vi "Spline_getPoint.vi"(8 "inputSPLINE":T1, 11 "Time":dbl) -> (3 "POSEwCURVATURE":T3={"CURVATURE"=0.0, "POSE"={"TRANSLATION"={"X"=0.0, "Y"=0.0}, "ROTATION"={"VALUE"=0.0, "COS"=1.0, "SIN"=0.0}}} {"POSE"."ROTATION"."SIN" format="%13.4f"; "POSE"."ROTATION"."COS" format="%13.4f"; "POSE"."ROTATION"."VALUE" format="%13.4f"; "POSE"."TRANSLATION"."Y" format="%14.3f"; "POSE"."TRANSLATION"."X" format="%14.3f"})   [LabVIEW 2019, in "Trajectory_Library.lvlib"]
doc: "Gets the pose and curvature at some point t on the spline.\n\nParameters:\n - Input Spline - Spline data structure\n - Time - The point in time to evaluate. (between 0 and 1)\n\nReturns:\n - PoseWCurve - The pose and curvature at that point."
uses:
  Trajectory_Library.lvlib
  TypeDef/POSEwCURVATURE.ctl
  TypeDef/POSE2D.ctl
  TypeDef/TRANSLATION2D.ctl
  TypeDef/ROTATION2D.ctl
  TypeDef/SPLINE.ctl
  <vilib>/Analysis/Matrix/Datatypes/RealMatrix.ctl
  <vilib>/Analysis/Matrix/Numeric/Multiply/Multiply - RM,RM.vi
  <vilib>/Analysis/Matrix/NI_Matrix.lvlib
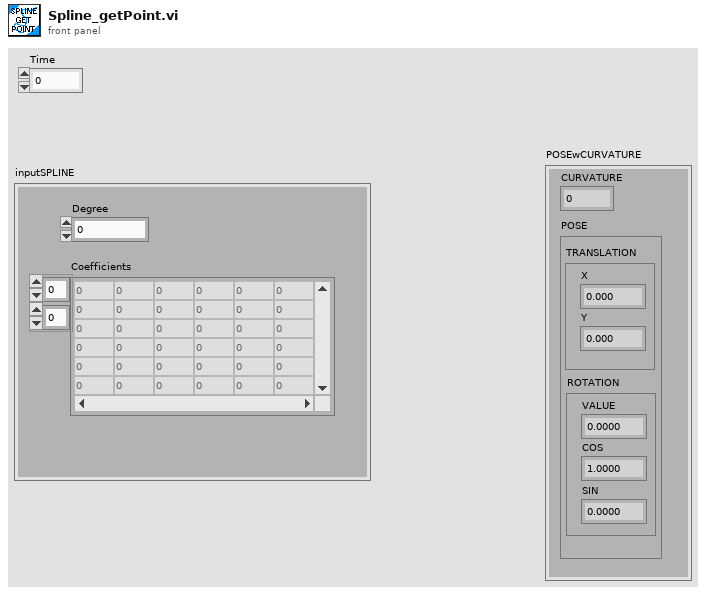
[diagram p1: front panel]
types:
  T1 = typedef "Trajectory_Library.lvlib/SPLINE.ctl" = cluster{"Degree":i32, "Coefficients":T2}
  T2 = typedef "NI_Matrix.lvlib/RealMatrix.ctl" = dbl[][]
  T3 = typedef "Trajectory_Library.lvlib/POSEwCURVATURE.ctl" = cluster{"CURVATURE":dbl, "POSE":T4}
  T4 = typedef "Trajectory_Library.lvlib/POSE2D.ctl" = cluster{"TRANSLATION":T5, "ROTATION":T6}
  T5 = typedef "Trajectory_Library.lvlib/TRANSLATION2D.ctl" = cluster{"X":dbl, "Y":dbl}
  T6 = typedef "Trajectory_Library.lvlib/ROTATION2D.ctl" = cluster{"VALUE":dbl, "COS":dbl, "SIN":dbl}
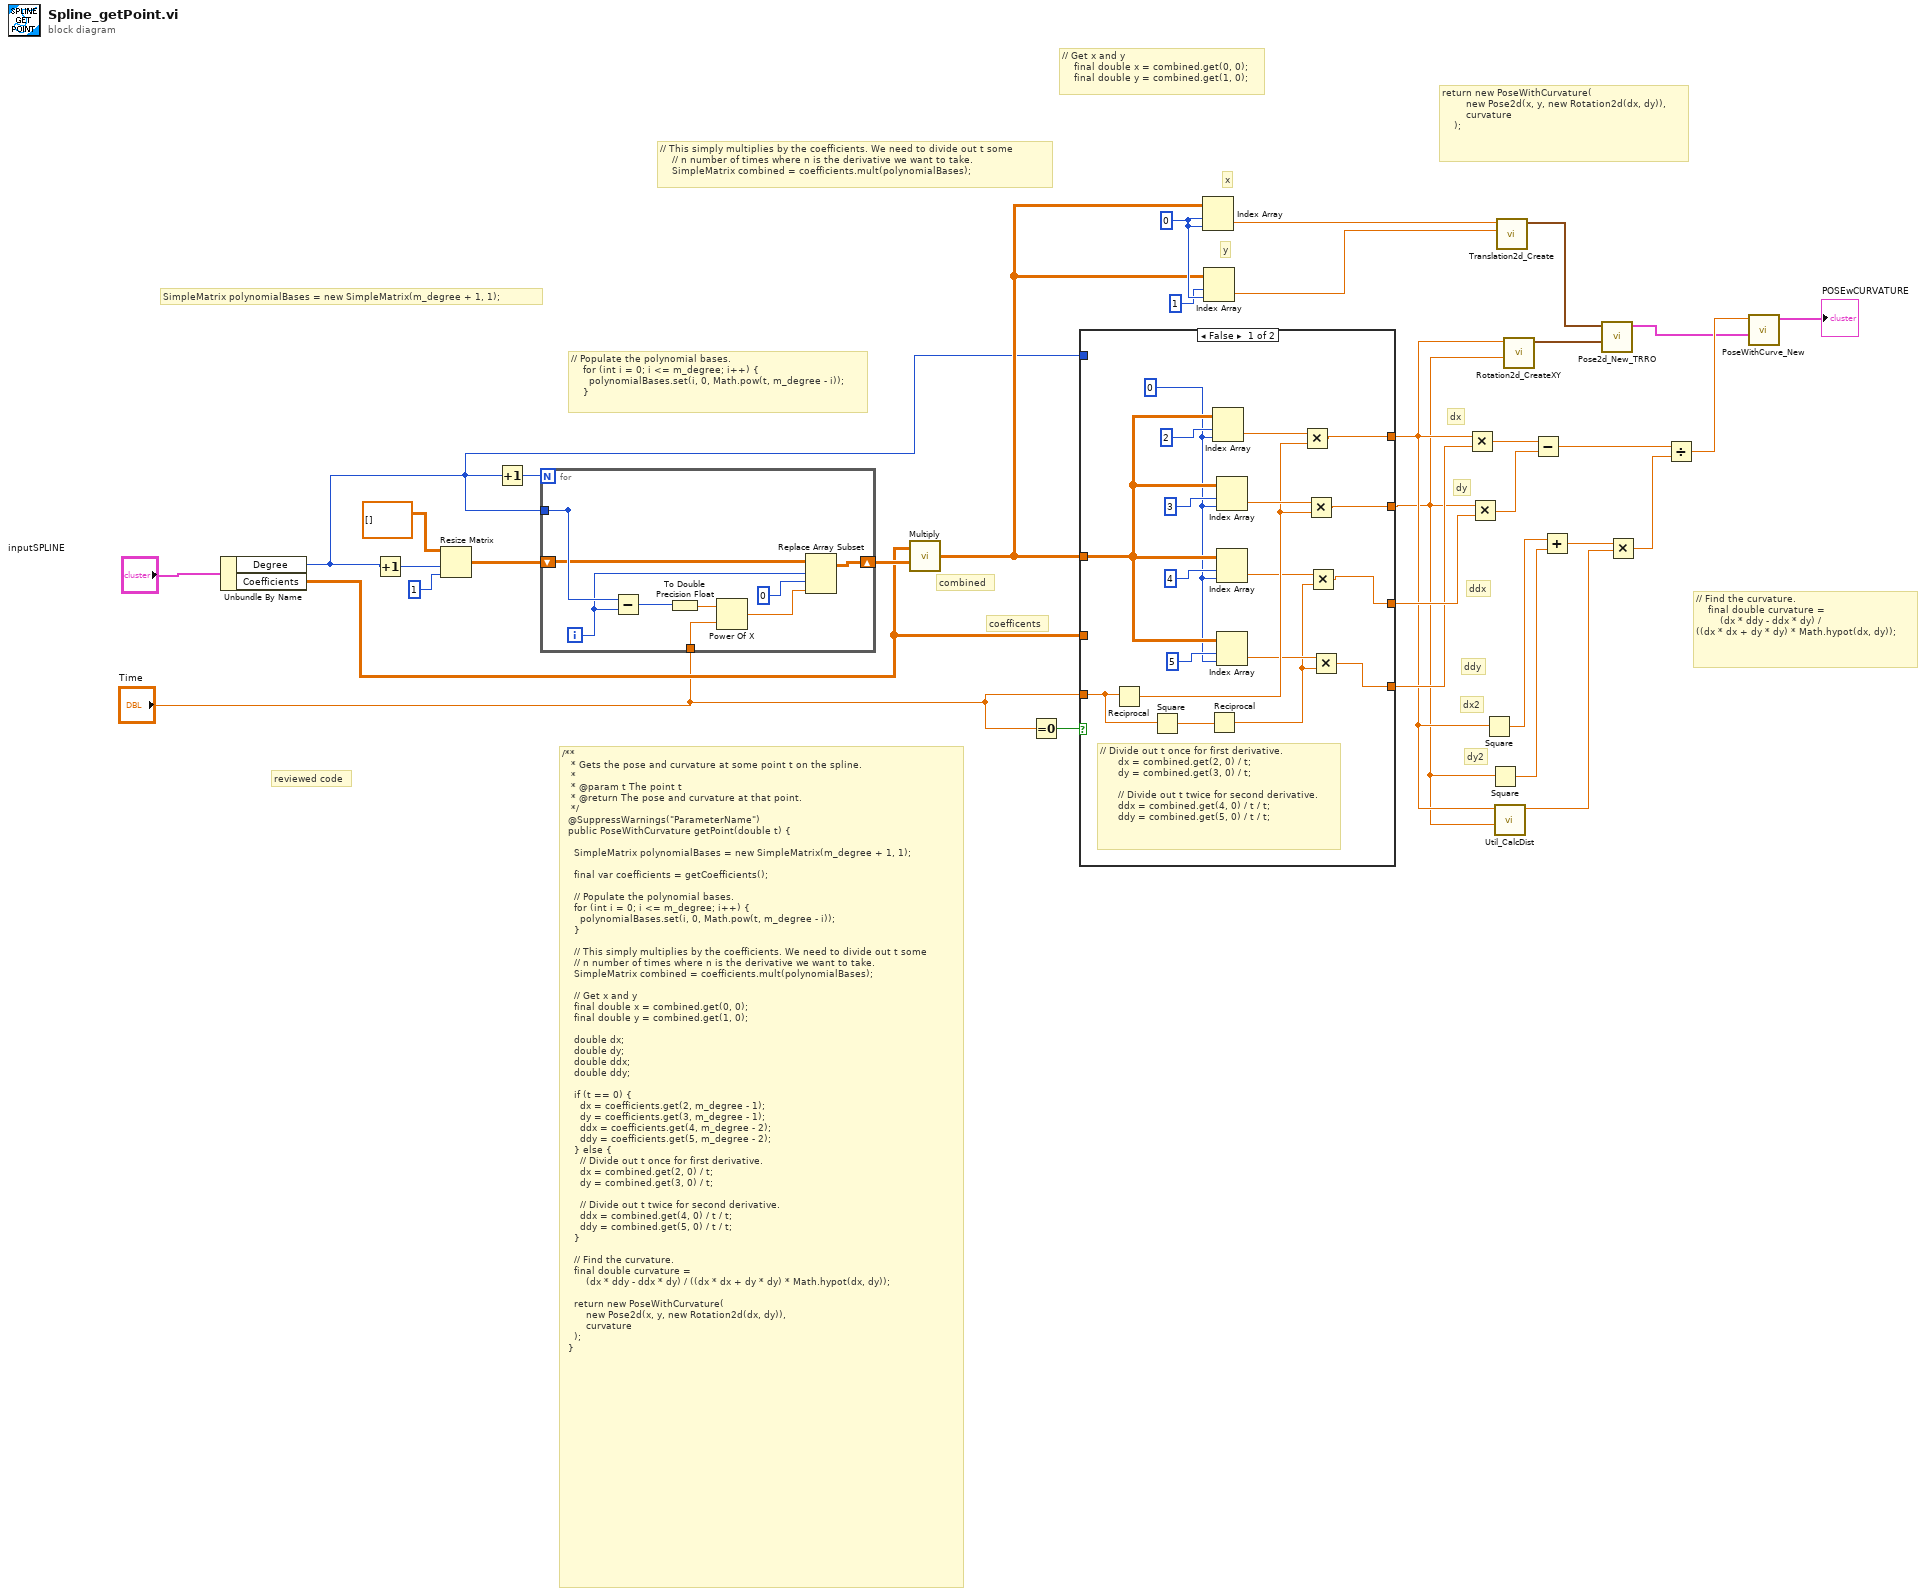
[diagram p0: block diagram]
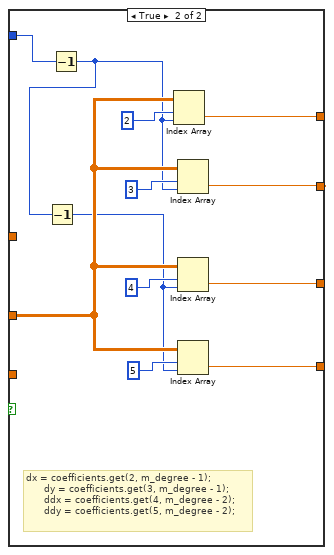
[diagram p2: hidden frame]
diagram:
  w27 = 0 ("index (row)")
  # "reviewed code"
  # "// Get x and y\n    final double x = combined.get(0, 0);\n    final double y = combined.get(1, 0);"
  # "// This simply multiplies by the coefficients. We need to divide out t some\n    // n number of times where n is the derivative we want to take.\n    SimpleMatrix combined = coefficients.mult(polynomialBases);"
  # "SimpleMatrix polynomialBases = new SimpleMatrix(m_degree + 1, 1);"
  # "return new PoseWithCurvature(\n        new Pose2d(x, y, new Rotation2d(dx, dy)),\n        curvature\n    );"
  # "dy2"
  # "dx2"
  # "// Find the curvature.\n    final double curvature =\n        (dx * ddy - ddx * dy) / \n((dx * dx + dy * dy) * Math.hypot(dx, dy));"
  # "ddy"
  # "ddx"
  # "dy"
  # "dx"
  # "coefficents"
  # "y"
  # "x"
  # "combined"
  # "// Populate the polynomial bases.\n    for (int i = 0; i <= m_degree; i++) {\n      polynomialBases.set(i, 0, Math.pow(t, m_degree - i));\n    }"
  # "/**\n   * Gets the pose and curvature at some point t on the spline.\n   *\n   * @param t The point t\n   * @return The pose and curvature at that point.\n   */\n  @SuppressWarnings(\"ParameterName\")\n  public PoseWithCurvature getPoint(double t) {\n\n    SimpleMatrix polynomialBases = new SimpleMatrix(m_degree + 1, 1);\n\n    final var coefficients = getCoefficients();\n\n    // Populate the polynomial bases.\n    for (int i = 0; i <= m_degree; i++) {\n      polynomialBases.set(i, 0, Math.pow(t, m_degree - i));\n    }\n\n    // This simply multiplies by the coefficients. We need to divide out t some\n    // n number of times where n is the derivative we want to take.\n    SimpleMatrix combined = coefficients.mult(polynomialBases);\n\n    // Get x and y\n    final double x = combined.get(0, 0);\n    final double y = combined.get(1, 0);\n\n    double dx;\n    double dy;\n    double ddx;\n    double ddy;\n\n    if (t == 0) {\n      dx = coefficients.get(2, m_degree - 1);\n      dy = coefficients.get(3, m_degree - 1);\n      ddx = coefficients.get(4, m_degree - 2);\n      ddy = coefficients.get(5, m_degree - 2);\n    } else {\n      // Divide out t once for first derivative.\n      dx = combined.get(2, 0) / t;\n      dy = combined.get(3, 0) / t;\n\n      // Divide out t twice for second derivative.\n      ddx = combined.get(4, 0) / t / t;\n      ddy = combined.get(5, 0) / t / t;\n    }\n\n    // Find the curvature.\n    final double curvature =\n        (dx * ddy - ddx * dy) / ((dx * dx + dy * dy) * Math.hypot(dx, dy));\n\n    return new PoseWithCurvature(\n        new Pose2d(x, y, new Rotation2d(dx, dy)),\n        curvature\n    );\n  }"
  n1 = Unbundle By Name("inputSPLINE") -> ("Degree"=w2:i32, "Coefficients"=w23:T2)
  n2 = Increment(x=w2) -> (x+1=w31:i32)
  n3 = Resize Matrix(1:1 ("number of columns"), 2:w31, 4:T2 [] ("matrix")) -> (0:w29:T2)
  n4 = Increment(x=w2) -> (x+1=w1:i32)
  n5 = for {
    N: w1 -> [_]
    shift-right: [w40] -> w25
    shift-left: w29 -> [w41]
    tunnel: [w42] -> _
    tunnel: w2 -> [w42]
    tunnel: "Time" -> [w36]
    i -> [w39]
    n6 = Subtract(x=w42, y=w39) -> (x-y=w35:i32)
    n7 = To Double Precision Float(number=w35) -> (double precision float=w34:dbl)
    n8 = Power Of X(1:w36, 2:w34) -> (0:w37:dbl)
    n9 = Replace Array Subset(array=w41, new element=w37, index (row)=w39, index (col)=0 ("disabled index (col)")) -> (w40:T2)
  }
  n10 = call-poly <vilib>:"Multiply.vi"("Real Matrix B"=w25, "Real Matrix A"=w23) -> ("A * B"=w24:T2)
  n11 = Equal To 0?(x="Time") -> (x = 0?=w28:bool)
  n12 = case shown="False" w28 {
    tunnel: w24 -> [w56 _]
    tunnel: w23 -> [_ w66]
    tunnel: w2 -> [_ w72]
    tunnel: [w49 w70] -> w5
    tunnel: [w48 w63] -> w4
    tunnel: [w47 w62] -> w22
    tunnel: [w46 w61] -> w19
    tunnel: "Time" -> [w45 _]
    frame False {
      w55 = 0
      # "// Divide out t once for first derivative.\n      dx = combined.get(2, 0) / t;\n      dy = combined.get(3, 0) / t;\n\n      // Divide out t twice for second derivative.\n      ddx = combined.get(4, 0) / t / t;\n      ddy = combined.get(5, 0) / t / t;"
      n13 = Reciprocal(x=w45) -> (1/x=w52:dbl)
      n14 = Square(x=w45) -> (x^2=w44:dbl)
      n15 = Reciprocal(x=w44) -> (1/x=w43:dbl)
      n16 = Index Array(array=w56, index (row)=2, index (col)=w55) -> (element=w54:dbl)
      n17 = Index Array(array=w56, index (row)=3, index (col)=w55) -> (element=w53:dbl)
      n18 = Index Array(array=w56, index (row)=4, index (col)=w55) -> (element=w51:dbl)
      n19 = Index Array(array=w56, index (row)=5, index (col)=w55) -> (element=w50:dbl)
      n20 = Multiply(x=w54, y=w52) -> (x*y=w49:dbl)
      n21 = Multiply(x=w53, y=w52) -> (x*y=w48:dbl)
      n22 = Multiply(x=w51, y=w43) -> (x*y=w47:dbl)
      n23 = Multiply(x=w50, y=w43) -> (x*y=w46:dbl)
    }
    frame True {
      # "dx = coefficients.get(2, m_degree - 1);\n      dy = coefficients.get(3, m_degree - 1);\n      ddx = coefficients.get(4, m_degree - 2);\n      ddy = coefficients.get(5, m_degree - 2);"
      n24 = Decrement(x=w72) -> (x-1=w65:i32)
      n25 = Decrement(x=w65) -> (x-1=w64:i32)
      n26 = Index Array(array=w66, index (row)=2, index (col)=w65) -> (element=w70:dbl)
      n27 = Index Array(array=w66, index (row)=3, index (col)=w65) -> (element=w63:dbl)
      n28 = Index Array(array=w66, index (row)=4, index (col)=w64) -> (element=w62:dbl)
      n29 = Index Array(array=w66, index (row)=5, index (col)=w64) -> (element=w61:dbl)
    }
  }
  n30 = Index Array(array=w24, index (row)=w27, index (col)=w27) -> (element=w14:dbl)
  n31 = Index Array(array=w24, index (row)=1, index (col)=w27) -> (element=w13:dbl)
  n32 = Multiply(x=w5, y=w19) -> (x*y=w21:dbl)
  n33 = Multiply(x=w4, y=w22) -> (x*y=w20:dbl)
  n34 = Square(x=w5) -> (x^2=w17:dbl)
  n35 = Square(x=w4) -> (x^2=w18:dbl)
  n36 = call "Util_CalcDist.vi"("Y"=w4, "X"=w5) -> ("DIST"=w3:dbl)  [unwired: 9 in]
  n37 = call "Translation2d_Create.vi"("Y"=w13, "X"=w14) -> ("TRANSLATION"=w12:T5)  [unwired: 9 in]
  n38 = call "Rotation2d_CreateXY.vi"("Y or sine"=w4, "X or  cosine"=w5) -> ("ROTATION"=w11:T6)  [unwired: 9 in]
  n39 = Subtract(x=w21, y=w20) -> (x-y=w16:dbl)
  n40 = Add(x=w17, y=w18) -> (x+y=w9:dbl)
  n41 = call "Pose2d_New_TRRO.vi"("ROTATION"=w11, "TRANSLATION"=w12) -> ("outPOSE"=w7:T4)  [unwired: 9 in]
  n42 = Multiply(x=w9, y=w3) -> (x*y=w15:dbl)
  n43 = Divide(x=w16, y=w15) -> (x/y=w8:dbl)
  n44 = call "PoseWithCurve_New.vi"("POSE"=w7, "CURVATURE"=w8) -> ("newPOSEwCURVATURE"=→"POSEwCURVATURE":T3)  [unwired: 9 in]
